vi "Add Global Request Handlers.vi"(11 "Request Handler Map In":T1) -> (3 "Request Handler Map":T1)   [LabVIEW 2020, in "HTTP Server.lvlib" / "Server.lvclass"]
uses:
  Server.lvclass
  PathValidation/PathValidation.lvclass
  Request Handler/Request Handler.lvclass
  Priority.ctl
  HTTP Server.lvlib
  Request Handler Map.ctl
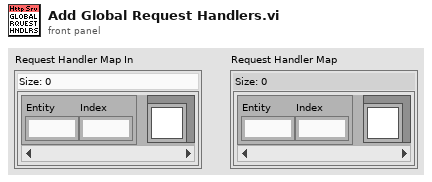
[diagram p1: front panel]
types:
  T1 = typedef "HTTP Server.lvlib/Request Handler Map.ctl" = map{T2, refnum<class "Request Handler.lvclass">}
  T2 = typedef "HTTP Server.lvlib/Priority.ctl" = cluster{"Entity":u16, "Index":u16}
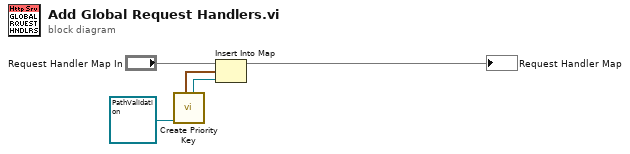
[diagram p0: block diagram]
diagram:
  n1 = call "Create Priority Key.vi"("Handler In"=refnum<class "PathValidation.lvclass"> refnum ("HTTP Server.lvlib:PathValidation.lvclass")) -> ("Handler"=w4:refnum<class "PathValidation.lvclass">, "Priority Key"=w5:T2)  [unwired: 8 in, 1 out]
  n2 = Insert Into Map(map in="Request Handler Map In", key=w5, value=w4) -> (map out=→"Request Handler Map":T1)  [unwired: 2 out]
